vi "ctx ap sync box query.vi"(7 "output_value":u32, 9 "cmd":u32(ring) items=["CAN_QUERY_CMD_GET_OUTPUT_PIN", "CAN_QUERY_CMD_GET_INPUT_PIN", "CAN_QUERY_CMD_GET_MODE", "CAN_QUERY_CMD_GET_LED_COLOR", "CAN_QUERY_CMD_GET_ERROR_STATE", "CAN_QUERY_CMD_GET_LAST_ERROR_STATE", "CAN_QUERY_CMD_GET_PCB_VERSION", "CAN_QUERY_CMD_GET_UID_LOW", "CAN_QUERY_CMD_GET_UID_MID", "CAN_QUERY_CMD_GET_UID_HIGH", "CAN_QUERY_CMD_GET_CAN_ERRORS", "CAN_QUERY_CMD_GET_OUTPUT_ERRORS", "CAN_QUERY_CMD_GET_INPUT_ERRORS", "CAN_QUERY_CMD_GET_FIRMWARE_VERSION", "CAN_QUERY_CMD_GET_LAST_ELEMENT"], 10 "ap_id":u32, 11 "context":u32) -> (2 "function return":i32, 3 "context out":u32, 5 "output_value out":u32)   [LabVIEW 2019, in "apdm.lvlib"]
doc: "APDM_EXPORT int apdm_ctx_ap_sync_box_query(apdm_ctx_t context, const uint32_t ap_id, const can_query_cmd_t cmd, uint32_t *output_value);"
uses:
  apdm.lvlib
  Lee Lab/CP FES Walking 2018/Code/Working/LabVIEW/apdm.dll
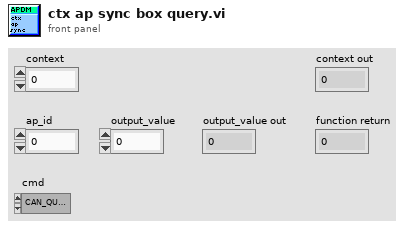
[diagram p1: front panel]
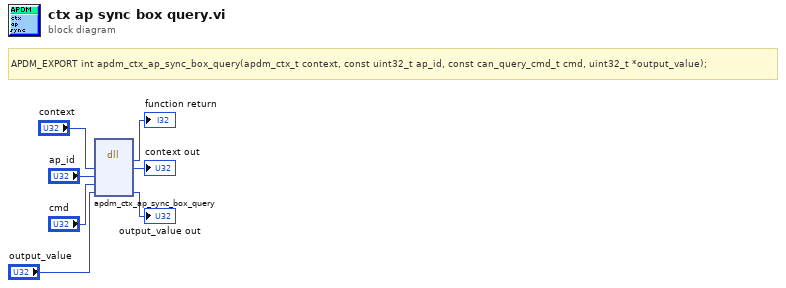
[diagram p0: block diagram]
diagram:
  # "APDM_EXPORT int apdm_ctx_ap_sync_box_query(apdm_ctx_t context, const uint32_t ap_id, const can_query_cmd_t cmd, uint32_t *output_value);"
  n1 = dll-call lib="C:/Users/jfalesi/Dropbox/Lee Lab/CP FES Walking 2018/Code/Working/LabVIEW/apdm.*" fn="apdm_ctx_ap_sync_box_query"("context"="context", "ap_id"="ap_id", "cmd"="cmd", "output_value"="output_value") -> (→"function return":i32, "context"=→"context out":u32, "output_value"=→"output_value out":u32)  [unwired: 5 in, 2 out]
